vi "Get Sender.vi"(8 "error in":errorcluster, 11 "CAN Message in":refnum<class "CAN Message.lvclass">) -> (0 "error out":errorcluster, 2 "Sender":string, 3 "CAN Message out":refnum<class "CAN Message.lvclass">)   [LabVIEW 2025, in "CAN Message.lvclass"]
uses:
  CAN Message.lvclass
  CAN Message.lvclass/CAN Message.ctl
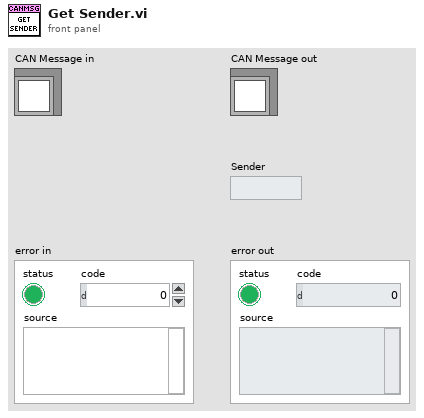
[diagram p1: front panel]
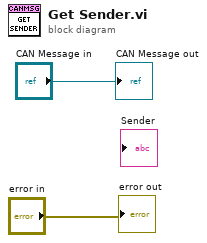
[diagram p0: block diagram]
diagram:
  "CAN Message out" <- "CAN Message in"
  "error out" <- "error in"
